vi "Stabilization.vi"(8 "error in (no error)":errorcluster, 9 "Stabilization\nInterval":dbl, 11 "Message Queues out":T2) -> (0 "error out":errorcluster)   [LabVIEW 2013, in "Timing and Stabilization.lvlib"]
uses:
  Timing and Stabilization.lvlib
  MeasurementControl Message Queue Folder/All Message Queues.ctl
  MeasurementControl Message Queue Folder/Message Cluster.ctl
  Stabilization.ctl
  Stabilization procedure select type def.ctl
  MeasurementControl Message Queue Folder/Enqueue Message (Single).vi
  MeasurementControl Message Queue Folder/MeasurementControl Message Queue.lvlib
panel:
  out "Stabilization Data":T1={"Stabilization waveform"={"t0"=timestamp(0 s since 1904-01-01), "dt"=50.0, "Y"=[10.0, 9.0, 8.75, 8.5, 8.25, 8.125, 8.06, 8.03, 8.015, 8.0, 8.0, 8.0]}, "Variation"=0.0, "Stabilized"=FALSE, "Threshold"=0.0, "time to stabilize"=0.0, "3 points"=[]}
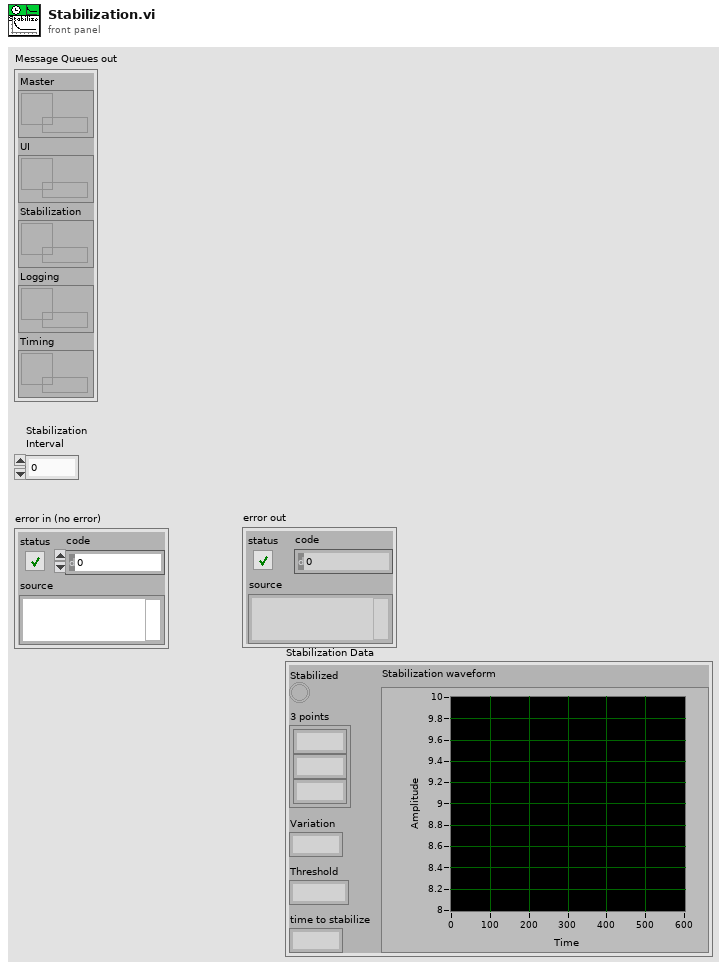
[diagram p1: front panel]
types:
  T1 = typedef "Timing and Stabilization.lvlib/Stabilization.ctl" = cluster{"Stabilization waveform":waveform(dbl), "Variation":dbl, "Stabilized":bool, "Threshold":dbl, "time to stabilize":dbl, "3 points":dbl[]}
  T2 = typedef "MeasurementControl Message Queue.lvlib/All Message Queues.ctl" = cluster{"Master":refnum<queue>, "UI":refnum<queue>, "Stabilization":refnum<queue>, "Logging":refnum<queue>, "Timing":refnum<queue>}
  T3 = typedef "Timing and Stabilization.lvlib/Stabilization procedure select type def.ctl" = enum16{"LM-79", "LM-51", "LM-9"}
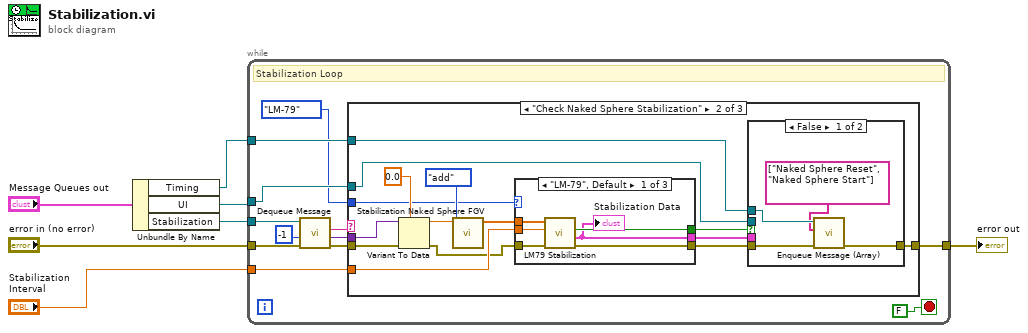
[diagram p0: block diagram]
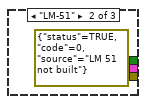
[diagram p3: hidden frame]
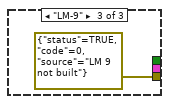
[diagram p4: hidden frame]
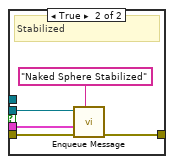
[diagram p5: hidden frame]
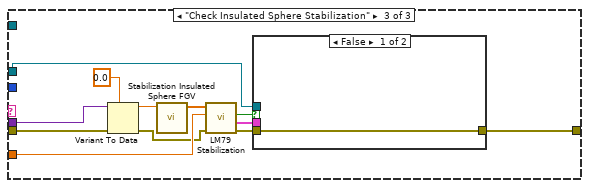
[diagram p6: hidden frame]
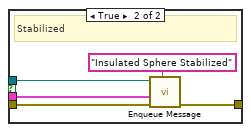
[diagram p7: hidden frame]
diagram:
  n1 = Unbundle By Name("Message Queues out") -> ("Timing"=w2:refnum<queue>, "UI"=w1:refnum<queue>, "Stabilization"=w5:refnum<queue>)
  n2 = while {
    tunnel: w5 -> [w17]
    tunnel: "Stabilization\nInterval" -> [w16]
    tunnel: w1 -> [w15]
    tunnel: w2 -> [w13]
    tunnel: [w9] -> w4
    tunnel: "error in (no error)" -> [w8]
    stop <- FALSE stop-if-true
    # "Stabilization Loop"
    n3 = call "Dequeue Message.vi"("error in (no error)"=w8, "timeout in ms (-1)"=-1, "Message Queue"=w17) -> ("error out"=w11:errorcluster, "Message Data"=w18:variant, "Message"=w19:string)  [unwired: 5 in, 1 out]
    n4 = case shown="\"Check Naked Sphere Stabilization\"" w19 {
      tunnel: w18 -> [_ w35 w64]
      tunnel: w16 -> [_ w31 w62]
      tunnel: w15 -> [_ w29 w60]
      tunnel: w13 -> [_ w26 _]
      tunnel: w11 -> [w20 w24 w54]
      tunnel: Stabilization_procedure_select_type_def."LM-79" -> [_ w22 _]
      tunnel: [w20 w21 w55] -> w9
      frame "False", Default {
      }
      frame "Check Naked Sphere Stabilization" {
        n5 = Variant To Data(error in=w24, type=0.0, Variant=w35) -> (data=w34:dbl, error out=w23:errorcluster)
        n6 = call "Stabilization Naked Sphere FGV.vi"("Control"=enum16{"reset", "add"}."add", "Stabilization Value In"=w34) -> ("Stabilization Array Out"=w32:dbl[])  [unwired: 9 in]
        n7 = case shown="\"LM-79\", Default" w22 {
          tunnel: w32 -> [w41 _ _]
          tunnel: w31 -> [w40 _ _]
          tunnel: [w39 errorcluster {"status"=TRUE, "code"=0, "source"="LM 51 not built"} ("error constant") errorcluster {"status"=TRUE, "code"=0, "source"="LM 9 not built"} ("error constant")] -> w30
          tunnel: [w36 _ _] -> w28
          tunnel: [w38 _ _] -> w27
          tunnel: w23 -> [w37 _ _]
          frame "LM-79", Default {
            n8 = call "LM79 Stabilization.vi"("error in (no error)"=w37, "Time Between\nMeasurements (s)"=w40, "Data over time"=w41) -> ("error out"=w39:errorcluster, "Stabilization Data"=w36:T1, "Stabilized"=w38:bool)  [unwired: 6 in]
            "Stabilization Data" <- w36
          }
          frame "LM-51" {
          }
          frame "LM-9" {
          }
        }
        n9 = case shown="False" w27 {
          tunnel: w30 -> [w45 w52]
          tunnel: w29 -> [_ w51]
          tunnel: w28 -> [_ w50]
          tunnel: w26 -> [w47 _]
          tunnel: [w44 w48] -> w21
          frame False {
            n10 = call "Enqueue Message (Array).vi"("error in (no error)"=w45, "Message Array"=string[] ["Naked Sphere Reset", "Naked Sphere Start"], "Message Queue"=w47) -> ("error out"=w44:errorcluster)  [unwired: 7 in, 1 out]
          }
          frame True {
            # "Stabilized"
            n11 = call-poly "Enqueue Message.vi"("error in (no error)"=w52, "Message Data"=w50, "Message"="Naked Sphere Stabilized", "Message Queue"=w51) -> ("error out"=w48:errorcluster)  [unwired: 6 in, 1 out]
          }
        }
      }
      frame "Check Insulated Sphere Stabilization" {
        n12 = Variant To Data(error in=w54, type=0.0, Variant=w64) -> (data=w57:dbl, error out=w53:errorcluster)
        n13 = call "Stabilization Insulated Sphere FGV.vi"("Stabilization Value In"=w57) -> ("Stabilization Array Out"=w56:dbl[])  [unwired: 10 in]
        n14 = call "LM79 Stabilization.vi"("error in (no error)"=w53, "Time Between\nMeasurements (s)"=w62, "Data over time"=w56) -> ("error out"=w61:errorcluster, "Stabilization Data"=w59:T1, "Stabilized"=w58:bool)  [unwired: 6 in]
        n15 = case shown="False" w58 {
          tunnel: w61 -> [w65 w70]
          tunnel: w60 -> [_ w69]
          tunnel: w59 -> [_ w68]
          tunnel: [w65 w66] -> w55
          frame False {
          }
          frame True {
            # "Stabilized"
            n16 = call-poly "Enqueue Message.vi"("error in (no error)"=w70, "Message Data"=w68, "Message"="Insulated Sphere Stabilized", "Message Queue"=w69) -> ("error out"=w66:errorcluster)  [unwired: 6 in, 1 out]
          }
        }
      }
    }
  }
  "error out" <- w4
